vi "Curtin_Tint.vi"(2 "Tint Factor":dbl=0.1 format="%#_13g", 3 "Plot.Plot Color":u32(colorbox)=16756242) -> (1 "Plot.Plot Color 2":u32(colorbox)=16756242)   [LabVIEW 2022 SP3]
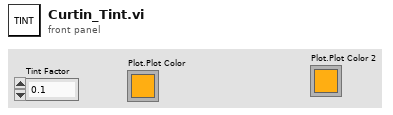
[diagram p1: front panel]
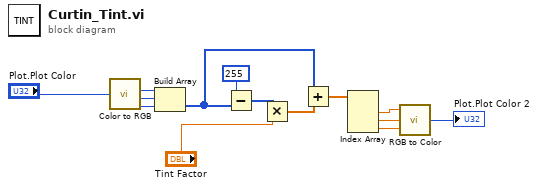
[diagram p0: block diagram]
diagram:
  n1 = call <vilib>:"Color to RGB.vi"("Color"="Plot.Plot Color") -> ("R"=w13:u8, "G"=w12:u8, "B"=w11:u8)  [unwired: 1 out]
  n2 = Build Array(w13, w12, w11) -> (w6:u8[])
  n3 = Subtract(x=u8 255, y=w6) -> (x-y=w9:u8[])
  n4 = Multiply(x=w9, y="Tint Factor") -> (x*y=w7:dbl[])
  n5 = Add(x=w6, y=w7) -> (x+y=w5:dbl[])
  n6 = Index Array(array=w5) -> (element #1=w4:dbl, element #2=w3:dbl, element #3=w2:dbl)  [unwired: 3 in]
  n7 = call <vilib>:"RGB to Color.vi"("B"=w2, "G"=w3, "R"=w4) -> ("Color"=→"Plot.Plot Color 2":u32)
